vi "TDC_addressDevice.vi"(8 "Error In":errorcluster, 11 "Device Number":i32) -> (0 "Error Out":errorcluster)   [LabVIEW 2011]
uses:
  tdcbase.dll
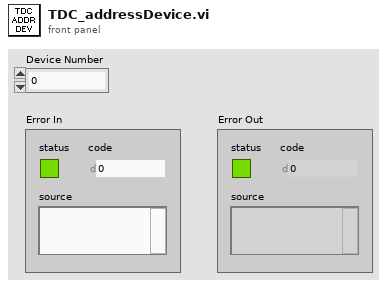
[diagram p1: front panel]
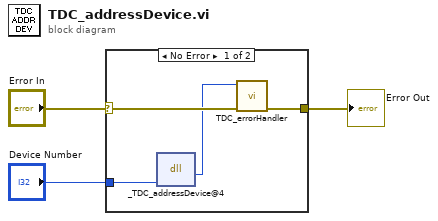
[diagram p0: block diagram]
diagram:
  n1 = case shown="No Error" "Error In" {
    selector: "Error In" -> [w7 w8]
    tunnel: [w6 w8] -> w2
    tunnel: "Device Number" -> [w4 _]
    frame No Error {
      n2 = dll-call lib="X:/tdcbase.dll" fn="_TDC_addressDevice@4"("devNo"=w4) -> ("return type"=w5:i32)  [unwired: 4 in, 2 out]
      n3 = call "TDC_errorHandler.vi"("Error In"=w7, "TDC Return Code"=w5) -> ("Error Out"=w6:errorcluster)  [unwired: 9 in]
    }
    frame Error {
    }
  }
  "Error Out" <- w2
